vi "Collect information from UI to run function.vi"(8 "error in (no error)":errorcluster, 11 "Function UI in":refnum<class "Controller UI.lvclass">) -> (0 "error out":errorcluster, 1 "Show UI?":bool, 2 "Devices":refnum<class "DevInfo.lvclass">[](array[class]), 3 "Function UI out":refnum<class "Controller UI.lvclass">, 4 "String":string, 5 "Function Name":string, 6 "Master?":bool)   [LabVIEW 2016, in "Controller UI.lvlib" / "Controller UI.lvclass"]
uses:
  <userlib>/Common Components/Controller UI/Controller UI.lvclass
  <userlib>/Common Components/Hardware/DevInfo/DevInfo.lvclass
  <userlib>/Common Components/Controller UI/Controller UI.lvclass/Controller UI.ctl
  <userlib>/Common Components/Hardware/DevInfo/DevInfo.lvclass/DevInfo.ctl
  <userlib>/Common Components/Hardware/DevInfo/Read Device Name.vi
  <userlib>/Common Components/Controller UI/Accessors/Read Function.vi
  <userlib>/Common Components/Controller UI/Accessors/Read Show FP_.vi
  <userlib>/Common Components/Controller UI/Accessors/Read Master_Slave.vi
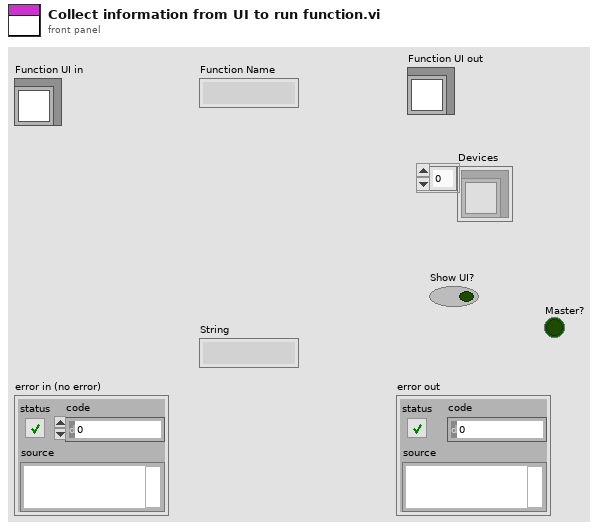
[diagram p1: front panel]
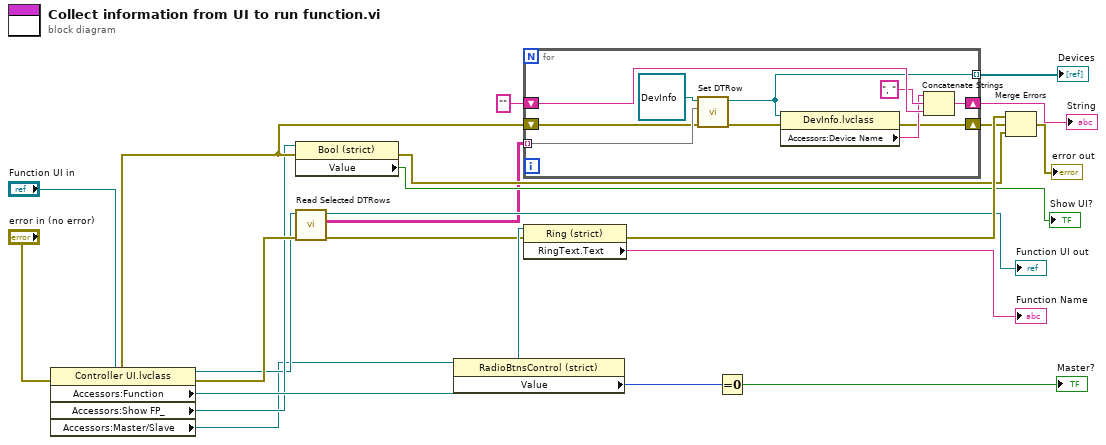
[diagram p0: block diagram]
diagram:
  n1 = property class="Controller UI.lvclass"(reference="Function UI in", error in="error in (no error)") -> (reference out=w7:refnum<class "Controller UI.lvclass">, error out=w16:errorcluster, "Accessors:Function"=w15:refnum<vi>, "Accessors:Show FP_"=w14:refnum<vi>, "Accessors:Master/Slave"=w3:refnum<vi>)
  n2 = property class="Bool (strict)"(reference=w14, error in="error in (no error)") -> (error out=w19:errorcluster, "Value"=→"Show UI?":bool)  [unwired: 1 out]
  n3 = call <userlib>:"Read Selected DTRows.vi"("error in (no error)"=w16, "Controller UI in"=w7) -> ("error out"=w8:errorcluster, "Selected DTRows"=w5:string[][], "Controller UI out"=→"Function UI out":refnum<class "Controller UI.lvclass">)  [unwired: 7 in]
  n4 = property class="RadioBtnsControl (strict)"(reference=w3) -> ("Value"=w2:enum32{"Master", "Slave"})  [unwired: 1 in, 2 out]
  n5 = for {
    shift-right: [w31] -> w12
    shift-left: "" -> [w30]
    shift-right: [w23] -> w18
    shift-left: "error in (no error)" -> [w24]
    tunnel: w5 -> [w28] mode=indexing
    tunnel: [w22] -> w4 mode=indexing
    n6 = call <userlib>:"Set DTRow.vi"("error in (no error)"=w24, "Dev Row Elements"=w28, "DevInfo in"=refnum<class "DevInfo.lvclass"> refnum ("Hardware.lvlib:DevInfo.lvclass")) -> ("error out"=w27:errorcluster, "DevInfo out"=w22:refnum<class "DevInfo.lvclass">)  [unwired: 7 in]
    n7 = property class="DevInfo.lvclass"(reference=w22, error in=w27) -> (error out=w23:errorcluster, "Accessors:Device Name"=w25:string)  [unwired: 1 out]
    n8 = Concatenate Strings(w25, ", " ("string"), w30) -> (w31:string)
  }
  "String" <- w12
  "Devices" <- w4
  n9 = property class="Ring (strict)"(reference=w15, error in=w8) -> (error out=w20:errorcluster, "RingText.Text"=→"Function Name":string)  [unwired: 1 out]
  n10 = Equal To 0?(x=w2) -> (x = 0?=→"Master?":bool)
  n11 = Merge Errors(w20, w18, w19) -> (→"error out":errorcluster)
